vi "focuswv.vi"(8 "frametime (s)":dbl, 9 "samplingrate":dbl=100.0) -> (0 "digwfs":digitalwaveform[](array[waveform]), 1 "YV":dbl[](array[numeric]), 2 "ZV":dbl[](array[numeric]), 3 "XV":dbl[](array[numeric]), 4 "samples":i32, 5 "dt":dbl)   [LabVIEW 2015]
uses:
  <vilib>/Waveform/DWDTOps.llb/DWDT Analog to Digital.vi
  <vilib>/measure/NI_MABase.lvlib
panel:
  out "x/y":dbl
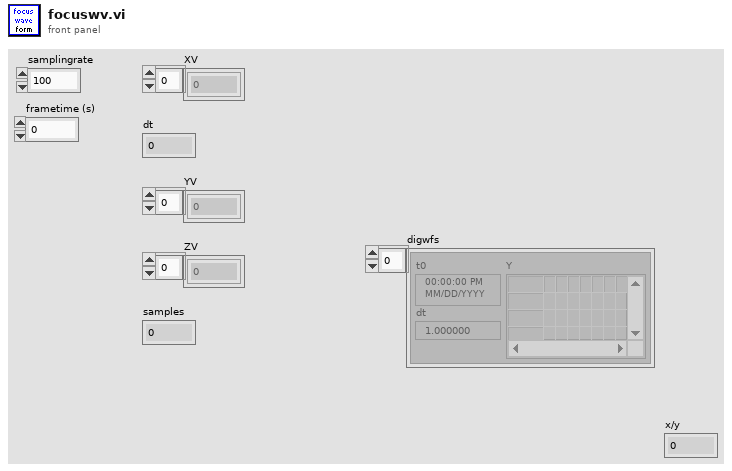
[diagram p1: front panel]
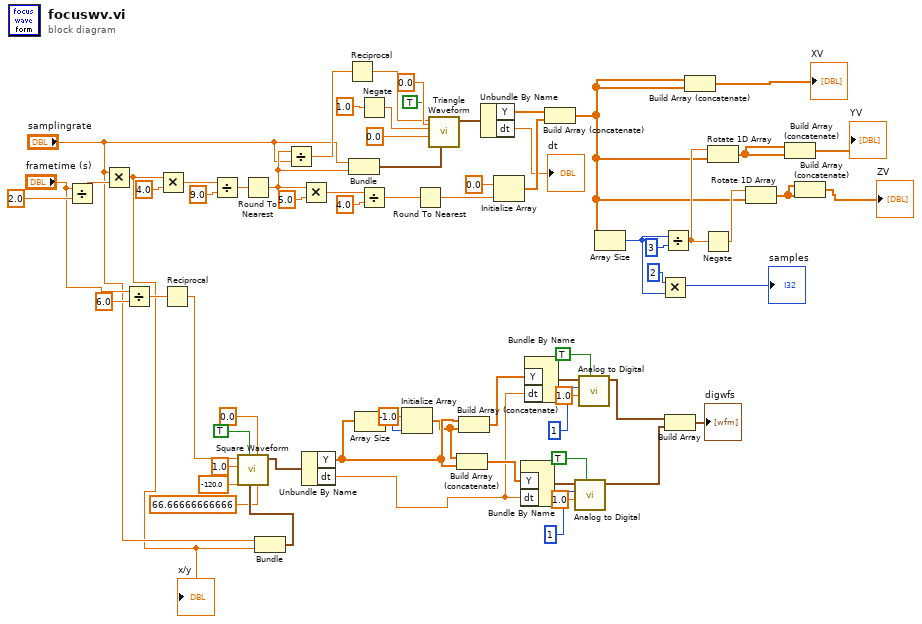
[diagram p0: block diagram]
diagram:
  n1 = Divide(x="frametime (s)", y=2.0) -> (x/y=w24:dbl)
  n2 = Multiply(x="samplingrate", y=w24) -> (x*y=w6:dbl)
  "x/y" <- w6
  n3 = Divide(x="frametime (s)", y=6.0) -> (x/y=w28:dbl)
  n4 = Multiply(x=w6, y=4.0) -> (x*y=w45:dbl)
  n5 = Reciprocal(x=w28) -> (1/x=w27:dbl)
  n6 = Divide(x=w45, y=9.0) -> (x/y=w47:dbl)
  n7 = Round To Nearest(number=w47) -> (nearest integer value=w55:dbl)
  n8 = Bundle("samplingrate"="samplingrate", w6) -> (w22:cluster{"samplingrate":dbl, dbl})  [unwired: 1 in]
  n9 = call <vilib>:"Square Waveform.vi"("duty cycle (%)"=66.66666666666, "offset"=0.0, "sampling info"=w22, "reset signal"=TRUE, "phase"=-120.0, "amplitude"=1.0, "frequency"=w27) -> ("signal out"=w20:waveform(dbl))  [unwired: 3 in, 1 out]
  n10 = Divide(x=w55, y="samplingrate") -> (x/y=w56:dbl)
  n11 = Multiply(x=w55, y=5.0) -> (x*y=w49:dbl)
  n12 = Unbundle By Name(w20) -> ("Y"=w17:dbl[], "dt"=w7:dbl)
  n13 = Reciprocal(x=w56) -> (1/x=w53:dbl)
  n14 = Bundle("samplingrate"="samplingrate", w55) -> (w51:cluster{"samplingrate":dbl, dbl})  [unwired: 1 in]
  n15 = Array Size(array=w17) -> (size(s)=w19:i32)
  n16 = Negate(x=1.0) -> (-x=w54:dbl)
  n17 = Divide(x=w49, y=4.0) -> (x/y=w61:dbl)
  n18 = Initialize Array(-1.0 ("element"), w19) -> (w16:dbl[])
  n19 = Round To Nearest(number=w61) -> (nearest integer value=w62:dbl)
  n20 = call <vilib>:"Triangle Waveform.vi"("offset"=0.0, "sampling info"=w51, "reset signal"=TRUE, "phase"=0.0, "amplitude"=w54, "frequency"=w53) -> ("signal out"=w63:waveform(dbl))  [unwired: 4 in, 1 out]
  n21 = Build Array (concatenate)(w16, w17) -> (w11:dbl[])
  n22 = Build Array (concatenate)(w17, w16) -> (w10:dbl[])
  n23 = Unbundle By Name(w63) -> ("Y"=w59:dbl[], "dt"=→"dt":dbl)
  n24 = Initialize Array(0.0 ("element"), w62) -> (w58:dbl[])
  n25 = Bundle By Name("Y"=w11, "dt"=w7) -> (w35:waveform(dbl))  [unwired: 1 in]
  n26 = Bundle By Name("Y"=w10, "dt"=w7) -> (w13:waveform(dbl))  [unwired: 1 in]
  n27 = Build Array (concatenate)(w59, w58) -> (w39:dbl[])
  n28 = call-poly <vilib>:"Analog to Digital.vi"("compress digital (T)"=TRUE, "full-scale range (pk-pk)"=1.0, "resolution (16 bit)"=1, "analog waveform"=w35) -> ("digital waveform"=w8:digitalwaveform)  [unwired: 4 in, 3 out]
  n29 = call-poly <vilib>:"Analog to Digital.vi"("compress digital (T)"=TRUE, "full-scale range (pk-pk)"=1.0, "resolution (16 bit)"=1, "analog waveform"=w13) -> ("digital waveform"=w9:digitalwaveform)  [unwired: 4 in, 3 out]
  n30 = Array Size(array=w39) -> (size(s)=w68:i32)
  n31 = Multiply(x=2, y=w68) -> (x*y=→"samples":i32)
  n32 = Divide(x=w68, y=3) -> (x/y=w66:dbl)
  n33 = Build Array(w9, w8) -> (→"digwfs":digitalwaveform[])
  n34 = Build Array (concatenate)(w39, w39) -> (→"XV":dbl[])
  n35 = Negate(x=w66) -> (-x=w67:dbl)
  n36 = Rotate 1D Array(1:w39, 2:w66) -> (0:w38:dbl[])
  n37 = Rotate 1D Array(1:w39, 2:w67) -> (0:w37:dbl[])
  n38 = Build Array (concatenate)(w38, w38) -> (→"YV":dbl[])
  n39 = Build Array (concatenate)(w37, w37) -> (→"ZV":dbl[])
